vi "5YJ556.vi"() -> ()   [LabVIEW 2015]
uses:
  <vilib>/DAQmx/read.llb/DAQmx Read (Analog 1D Wfm NChan NSamp).vi
  <vilib>/DAQmx/create/channels.llb/DAQmx Create Channel (AI-Bridge).vi
  <vilib>/DAQmx/configure/timing.llb/DAQmx Timing (Sample Clock).vi
  <vilib>/DAQmx/miscellaneous.llb/DAQmx Fill In Error Info.vi
panel:
  out "Numeric 4":dbl
  out "Numeric 3":dbl
  out "Numeric 2":dbl
  out "Numeric":dbl
  out "Waveform Chart 6":dynamicdata(graph)
  out "Waveform Chart 5":dynamicdata(graph)
  out "Waveform Chart 4":dynamicdata(graph)
  out "Waveform Chart 3":i32(graph)
  out "Filtered Signal":dbl
  out "data":waveform(dbl)[](array[waveform])
  in  "rate":dbl=1000.0 format="%0.2f"
  out "Waveform Chart 2":dynamicdata(graph)
  in  "Samples per Loop":i32=100
  out "array":dbl[](array[numeric])
  in  "stop":bool
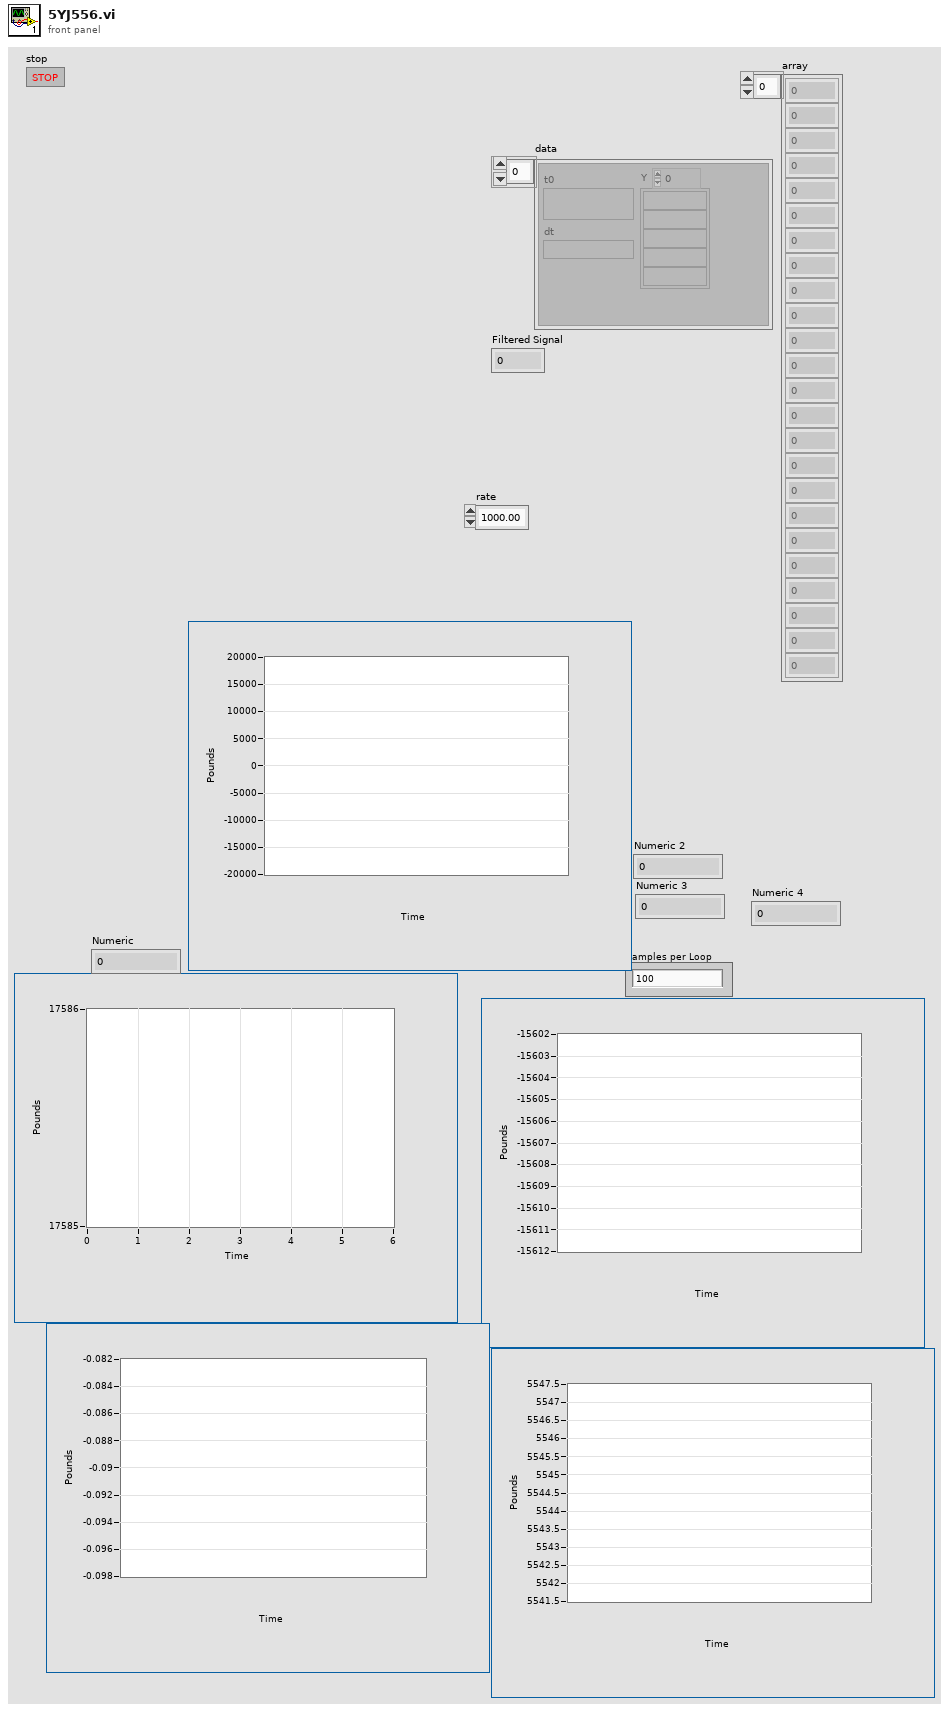
[diagram p1: front panel]
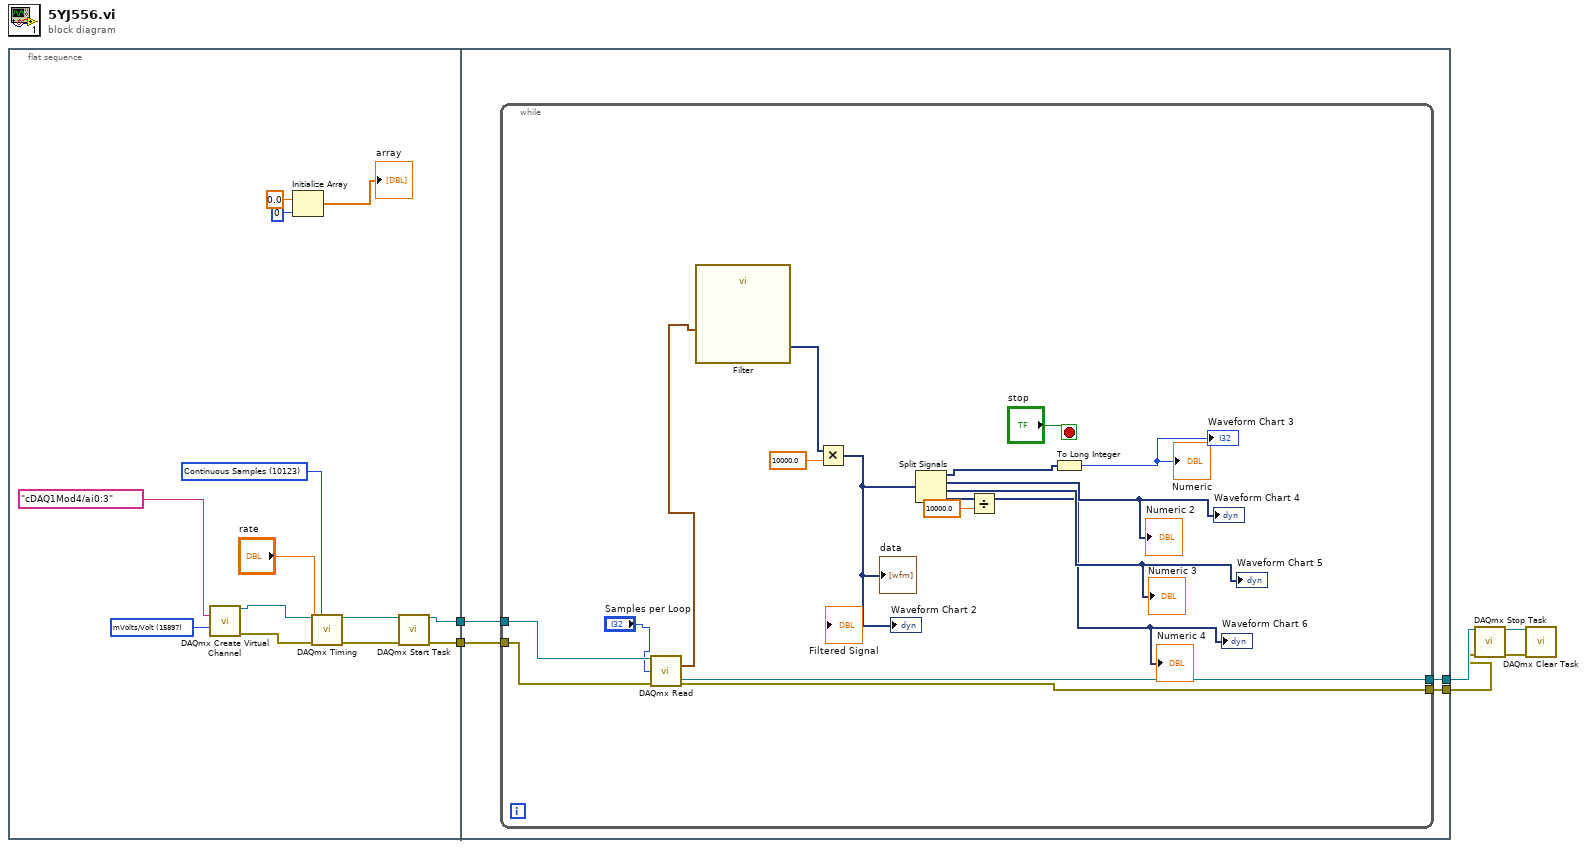
[diagram p0: block diagram]
diagram:
  n1 = flat-sequence {
    tunnel: [w16] -> w2
    tunnel: [w15] -> w1
    tunnel: [w23] -> w4
    tunnel: [w22] -> w3
    tunnel: w2 -> [w21]
    tunnel: w1 -> [w20]
    frame #0 {
      w7 = 15897 items=["Volts/Volt"=15896, "mVolts/Volt"=15897, "From Custom Scale"=10065] ("units")
      w12 = 10123 items=["Finite Samples"=10178, "Continuous Samples"=10123, "Hardware Timed Single Point"=12522] ("sample mode")
      n2 = call-poly <vilib>:"DAQmx Create Virtual Channel.vi"("physical channels"=tag "cDAQ1Mod4/ai0:3", "units"=w7) -> ("task out"=w11:refnum<k21>, "error out"=w10:errorcluster)  [unwired: 12 in]
      n3 = Initialize Array(0.0 ("element"), 0 ("dimension size")) -> (→"array":dbl[])
      n4 = call-poly <vilib>:"DAQmx Timing.vi"("task/channels in"=w11, "sample mode"=w12, "rate"="rate", "error in"=w10) -> ("task out"=w14:refnum<k21>, "error out"=w13:errorcluster)  [unwired: 10 in]
      n5 = call <vilib>:"DAQmx Start Task.vi"("task/channels in"=w14, "error in"=w13) -> ("task out"=w16:refnum<k21>, "error out"=w15:errorcluster)  [unwired: 12 in]
    }
    frame #1 {
      n6 = while {
        tunnel: [w39] -> w23
        tunnel: [w38] -> w22
        tunnel: w21 -> [w37]
        tunnel: w20 -> [w36]
        stop <- "stop" stop-if-true
        n7 = call-poly <vilib>:"DAQmx Read.vi"("task/channels in"=w37, "number of samples per channel"="Samples per Loop", "error in"=w36) -> ("task out"=w39:refnum<k21>, "data"=w34:waveform(dbl)[], "error out"=w38:errorcluster)  [unwired: 10 in]
        n8 = call "Filter"("Signal"=w34) -> ("Filtered Signal"=w32:dynamicdata)  [unwired: 9 in, 1 out]
        n9 = Multiply(x=w32, y=10000.0) -> (x*y=w31:dynamicdata)
        "Waveform Chart 2" <- w31
        "data" <- w31
        "Filtered Signal" <- w31
        n10 = Split Signals(w31) -> (w25:dynamicdata, →"Waveform Chart 4" →"Numeric 2":dynamicdata, →"Waveform Chart 5" →"Numeric 3":dynamicdata, w28:dynamicdata)  [unwired: 4 in]
        n11 = Divide(x=w28, y=10000.0) -> (x/y=→"Waveform Chart 6" →"Numeric 4":dynamicdata)
        n12 = To Long Integer(number=w25) -> (32bit integer=→"Waveform Chart 3" →"Numeric":i32)
      }
    }
  }
  n13 = call <vilib>:"DAQmx Stop Task.vi"("task/channels in"=w4, "error in"=w3) -> ("task out"=w6:refnum<k21>, "error out"=w5:errorcluster)  [unwired: 12 in]
  n14 = call <vilib>:"DAQmx Clear Task.vi"("task in"=w6, "error in"=w5) -> ()  [unwired: 13 in, 1 out]
